vi "Calibration.vi"(0 "Mode":T3, 5 "Calib file":path, 9 "Simulate/Run":T2) -> (14 "Calib const":string[][](array[string]), 16 "Coefficients":dbl[][](array[numeric]) format="%.2f", 19 "Status Out":T1)   [LabVIEW 2021]
uses:
  Anemometry Sub Vis/Calibration/Calib_mode.ctl
  Anemometry Sub Vis/Controls/User_Specific_mode.ctl
  Anemometry Sub Vis/Gen Trav/Multi_Run_Status.ctl
  Anemometry Sub Vis/Controls/Post_Process.ctl
  Anemometry Sub Vis/Globals/Calib_global.vi
  Anemometry Sub Vis/Globals/Meas_global.vi
panel:
  in  "-ve Ref Values":bool
  out "String":string
  in  "poly fit order":i32=2 caption="Polynomial\nOrder" min=1 max=4 step=1
  out "Ref velocity":dbl[](array[numeric])=[2.4275346736, 2.4395664609, 2.453235235, 2.4247395837, 2.4277603784, 2.41169823, 2.4254144559, 2.424896502176921] format="%.3f"
  out "labels":string[](array[string])=["XW1 Volt", "XW2 Volt", "Entered Val", "Selector"]
  in  "Point selector 3":cluster{"Y":dbl, "X":dbl, "t/f":bool}[](array[cluster]) {"X" format="%#.2g"; "Y" format="%#.3f"}
  in  "n":dbl=0.45 format="%.4f"
  in  "Fixed n":bool=TRUE
  out "Sample of input signals":dbl[][](graph)
  in  "Sampling speeds":T4={"Samples/ch"=600, "Sample Rate/ch (Hz)"=100.0} {"Sample Rate/ch (Hz)" min=0; "Samples/ch" min=0 step=1}
  out "Calibration plot":cluster{cluster{dbl, dbl}[]}[](graph)
  in  "Point selector 4":T5(array[cluster]) {"Y2" format="%#.2f"; "X" format="%#.3f"; "Y" format="%#.2f"}
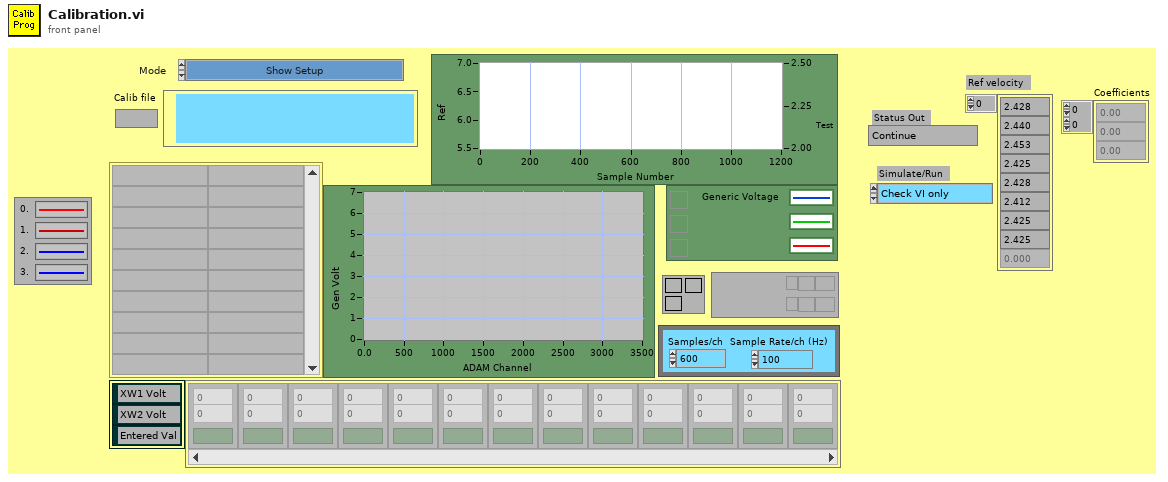
[diagram p1: front panel]
types:
  T1 = typedef "Multi_Run_Status.ctl" = enum16{"Continue", "Continue with Error", "Jump to Next Point", "Jump to Next Row", "Jump To Fall Back", "Terminate Run"}
  T2 = typedef "User_Specific_mode.ctl" = enum16{"Check VI only", "Run VI"}
  T3 = typedef "Calib_mode.ctl" = enum16{"Show Setup", "Take a New Calibration Point", "Refit Curve", "Setup Front Panel"}
  T4 = cluster{"Samples/ch":i32, "Sample Rate/ch (Hz)":sgl}
  T5 = cluster{"Y":dbl, "Y2":dbl, "X":dbl, "t/f":bool}[]
  T6 = typedef "Post_Process.ctl" = enum16{"Take New Data", "Post Process Raw Data File"}
  T7 = cluster{"Samples /ch":i32, "Sampling Rate /ch (Hz)":sgl}
  T8 = typedef "Ref_Inst_type.ctl" = enum16{"Propellor anemometer", "Pressure Transducer", "Raw voltage", "Pitot-static tube", "Generic Linear", "Generic Polynomial", "Thermocouple", "LDA", "Enter Value", "ADAM Channel"}
  T9 = typedef "Cal_Inst_type.ctl" = enum16{"Propeller anemometer", "Pressure Transducer", "Hot wire", "Cross wire velocity", "Cross wire angle", "Generic Linear", "Generic Polynomial", "Poly Fit Special", "Fast FID", "Thermocouple", "Cold wire", "Pulsed Wire"}
  T10 = cluster{"2nd Ref type":T8, "2nd inst present":bool}
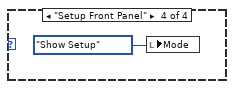
[diagram p4: hidden frame]
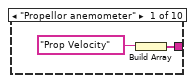
[diagram p8: hidden frame]
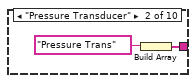
[diagram p9: hidden frame]
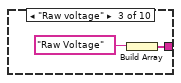
[diagram p10: hidden frame]
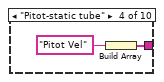
[diagram p11: hidden frame]
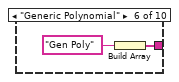
[diagram p12: hidden frame]
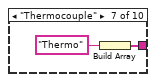
[diagram p13: hidden frame]
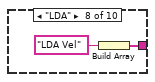
[diagram p14: hidden frame]
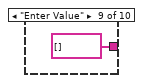
[diagram p15: hidden frame]
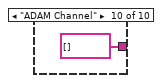
[diagram p16: hidden frame]
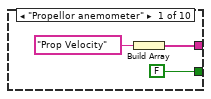
[diagram p17: hidden frame]
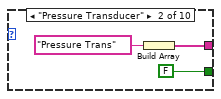
[diagram p18: hidden frame]
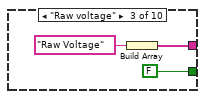
[diagram p19: hidden frame]
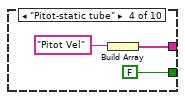
[diagram p20: hidden frame]
diagram:
  # "Temporary error bus for flow\ncontrol. No errors ever get\nwritten to it."
  n1 = flat-sequence {
    tunnel: "Simulate/Run" -> [w46]
    tunnel: errorcluster {"status"=FALSE, "code"=0, "source"=""} ("error constant") -> [w42]
    tunnel: [w42] -> w18
    frame #0 {
      w44 = FALSE  # Visible
      # "Calibration-Frame0"
      n2 = call "Run_EnFlo_Hub.vi"() -> ()  [unwired: 1 in, 7 out]
      n3 = case shown="\"Run VI\"" w46 {
        frame "Check VI only" {
        }
        frame "Run VI" {
          n4 = Current VI's Path() -> (path=w48:path)
          n5 = call "Open_Close_Front_Panel.ph.vi"("openWindow (T)"=TRUE ("Front Panel Window:Open"), "VI path"=w48) -> ()  [unwired: 1 in, 1 out]
        }
      }
      n6 = property on="String" class="Str"("Visible"=w44, "Blinking"=w44) -> ()  [unwired: 2 in, 2 out]
      n7 = global write "Calib_global.vi" "New Setup String"("") -> ()
      n8 = global write "Meas_global.vi" "Raw data option"(enum16{"Save raw data", "Raw data not saved"}."Save raw data" ("Raw data option")) -> ()
      n9 = global write "Meas_global.vi" "Post Process"(Post_Process."Take New Data" ("Post Process")) -> ()
    }
  }
  n10 = flat-sequence {
    tunnel: [w55] -> w2
    tunnel: [w54] -> w22
    tunnel: [w53] -> w38
    tunnel: w18 -> [w51]
    tunnel: [w51] -> w17
    tunnel: "Mode" -> [w50]
    frame #0 {
      # "Calibration-Frame1"
      n11 = call "Cal1-GetPath.vi"("Mode in"=w50, "Calib file"="Calib file") -> ("String output"=w53:string, "exists?"=w55:bool, "Path output"=w54:path)  [unwired: 7 in]
      n12 = local write "Calib file"(w54) -> ()
    }
  }
  n13 = flat-sequence {
    tunnel: [w63] -> w21
    tunnel: w22 -> [w62]
    tunnel: [w61] -> w36
    tunnel: [w60] -> w20
    tunnel: w17 -> [w59]
    tunnel: [w59] -> w16
    tunnel: "Mode" -> [w56]
    frame #0 {
      # "Calibration-Frame2"
      n14 = Current VI's Path() -> (path=w58:path)
      n15 = call "Running_as_top_level.vi"("Vi path name"=w58) -> ("Top Level"=w57:bool)  [unwired: 1 out]
      n16 = call "Cal2-GetMode.vi"("Calibration.vi running as top level VI?"=w57, "Mode in"=w56, "Path in"=w62) -> ("data mode"=w63:enum16{"Take new data point", "Refit Curve"}, "Mode out"=w60:T3, "Boolean"=w61:bool)  [unwired: 6 in]
    }
  }
  n17 = flat-sequence {
    tunnel: w21 -> [w68]
    tunnel: w20 -> [w67]
    tunnel: w36 -> [w65]
    tunnel: w16 -> [w64]
    tunnel: [w64] -> w15
    frame #0 {
      # "Calibration-Frame3"
      n18 = local read "Fixed n"() -> (w70:bool)
      n19 = call "Cal3-GetSetup.vi"("Sampling speeds"="Sampling speeds", "data mode"=w68, "Fixed n"=w70, "Mode in"=w67, "Boolean in"=w65) -> ("Sampling speeds Output"=w71:T7, "Fixed n out"=w69:bool, "Boolean out"=w66:bool)  [unwired: 4 in]
      n20 = case shown="True" w66 {
        tunnel: w71 -> [_ w74]
        tunnel: w69 -> [_ w73]
        frame False {
        }
        frame True {
          n21 = local write "Sampling speeds"(w74) -> ()
          n22 = local write "Fixed n"(w73) -> ()
        }
      }
    }
  }
  n23 = flat-sequence {
    tunnel: [w81] -> w39
    tunnel: [w80] -> w40
    tunnel: w22 -> [w79]
    tunnel: w2 -> [w78]
    tunnel: w38 -> [w77]
    tunnel: w15 -> [w76]
    tunnel: [w76] -> w14
    tunnel: "Mode" -> [w75]
    frame #0 {
      # "Calibration-Frame4"
      n24 = case shown="\"Setup Front Panel\"" w75 {
        frame Default {
        }
        frame "Setup Front Panel" {
          n25 = global read "Calib_global.vi" "Pre Setup String"() -> (w83:string)
          n26 = call "Get_value_from_string.vi"("Input string"=w83, "Variable name"="Polynomial Fit Order" ("Label for value")) -> ("Value"=w82:dbl)  [unwired: 1 in, 1 out]
          n27 = local write "poly fit order"(w82) -> ()
        }
      }
      n28 = call "Cal4-GetCalDataFrFile.vi"("StringName"=w77, "FileExists?"=w78, "CalibFilePath"=w79) -> ("CalibData"=w81:string, "HasData"=w80:bool)  [unwired: 7 in]
    }
  }
  n29 = flat-sequence {
    tunnel: w14 -> [w85]
    tunnel: [w85] -> w13
    frame #0 {
      w88 = ""
      # "Calibration-Frame5"
      n30 = global read "Calib_global.vi" "Ref Instrument type"() -> (w96:T8)
      n31 = global read "Calib_global.vi" "Instrument type"() -> (w99:T9)
      n32 = global read "Calib_global.vi" "2nd ref instrument"() -> (w95:T10)
      n33 = case shown="\"Generic Linear\"" w96 {
        tunnel: [w123 w126 w130 w132 w135 w138 w141 w144 string[] [] string[] []] -> w92
        tunnel: [FALSE FALSE FALSE FALSE FALSE FALSE FALSE FALSE FALSE FALSE] -> w87
        frame "Propellor anemometer" {
          n34 = Build Array("Prop Velocity") -> (w123:string[])
        }
        frame "Pressure Transducer" {
          n35 = Build Array("Pressure Trans") -> (w126:string[])
        }
        frame "Raw voltage" {
          n36 = Build Array("Raw Voltage") -> (w130:string[])
        }
        frame "Pitot-static tube" {
          n37 = Build Array("Pitot Vel") -> (w132:string[])
        }
        frame "Generic Linear" {
          n38 = Build Array("Gen Lin") -> (w135:string[])
        }
        frame "Generic Polynomial" {
          n39 = Build Array("Gen Poly") -> (w138:string[])
        }
        frame "Thermocouple" {
          n40 = Build Array("Thermo") -> (w141:string[])
        }
        frame "LDA" {
          n41 = Build Array("LDA Vel") -> (w144:string[])
        }
        frame "Enter Value" {
        }
        frame "ADAM Channel" {
        }
      }
      n42 = case shown="\"Thermocouple\"" w99 {
        tunnel: [w154 w158 w162 w166 w171 w176 w180 w184 w188 w192 w196 w201] -> w89
        tunnel: [FALSE FALSE FALSE FALSE FALSE FALSE TRUE TRUE FALSE FALSE TRUE TRUE] -> w91
        tunnel: [w152 w156 w160 w164 w169 w174 w178 w182 w186 w190 w194 FALSE] -> w86
        tunnel: w87 -> [w152 w156 w160 w164 w169 w174 w178 w182 w186 w190 w194 _]
        frame "Propeller anemometer" {
          n43 = Build Array("Prop Voltage") -> (w154:string[])
        }
        frame "Pressure Transducer" {
          n44 = Build Array("Pressure Trans") -> (w158:string[])
        }
        frame "Hot wire" {
          n45 = Build Array("HW Voltage") -> (w162:string[])
        }
        frame "Cross wire velocity" {
          n46 = Build Array("XW1 Voltage", "XW2 Voltage") -> (w166:string[])
        }
        frame "Cross wire angle" {
          n47 = Build Array("XW1 Voltage", "XW2 Voltage") -> (w171:string[])
        }
        frame "Generic Linear" {
          n48 = Build Array("Generic Voltage") -> (w176:string[])
        }
        frame "Generic Polynomial" {
          n49 = Build Array("Generic Voltage") -> (w180:string[])
        }
        frame "Poly Fit Special" {
          n50 = Build Array("Generic Voltage") -> (w184:string[])
        }
        frame "Fast FID" {
          n51 = Build Array("FF Voltage") -> (w188:string[])
        }
        frame "Thermocouple" {
          n52 = Build Array("Thermo Voltage") -> (w192:string[])
        }
        frame "Cold wire" {
          n53 = Build Array("CW Voltage") -> (w196:string[])
        }
        frame "Pulsed Wire" {
          n54 = local write "poly fit order"(3 ("polynomial order")) -> ()
          n55 = Build Array("PWA 1/TOF") -> (w201:string[])
        }
      }
      n56 = Unbundle By Name(w95) -> ("2nd Ref type"=w93:T8, "2nd inst present"=w94:bool)
      n57 = case shown="True" w94 {
        tunnel: w93 -> [_ w102]
        tunnel: [w101 w103] -> w90
        tunnel: w92 -> [w101 _]
        frame False {
        }
        frame True {
          n58 = case shown="\"Generic Linear\"" w102 {
            tunnel: [w104 w106 w109 w110 w112 w114 w116 w118 string[] [] string[] []] -> w103
            frame "Propellor anemometer" {
              n59 = Build Array("Prop Velocity") -> (w104:string[])
            }
            frame "Pressure Transducer" {
              n60 = Build Array("Pressure Trans") -> (w106:string[])
            }
            frame "Raw voltage" {
              n61 = Build Array("Raw Voltage") -> (w109:string[])
            }
            frame "Pitot-static tube" {
              n62 = Build Array("Pitot Vel") -> (w110:string[])
            }
            frame "Generic Linear" {
              n63 = Build Array("Gen Lin") -> (w112:string[])
            }
            frame "Generic Polynomial" {
              n64 = Build Array("Gen Poly") -> (w114:string[])
            }
            frame "Thermocouple" {
              n65 = Build Array("Thermo") -> (w116:string[])
            }
            frame "LDA" {
              n66 = Build Array("LDA Vel") -> (w118:string[])
            }
            frame "Enter Value" {
            }
            frame "ADAM Channel" {
            }
          }
        }
      }
      n67 = case shown="False" w86 {
        frame False {
          n68 = local write "-ve Ref Values"(FALSE ("-ve Ref Values")) -> ()
        }
        frame True {
        }
      }
      n69 = Build Array (concatenate)(w90, w89, w88, w88, w88) -> (w97:string[])
      n70 = property on="-ve Ref Values" class="Bool (strict)"("Visible"=w86) -> ()  [unwired: 2 in, 2 out]
      n71 = property on="poly fit order" class="DigNum (strict)"("Visible"=w91) -> ()  [unwired: 2 in, 2 out]
      n72 = for {
        N: 3 -> [_]
        tunnel: w97 -> [w150] mode=indexing
        i -> [w151]
        n73 = property on="Sample of input signals" class="WFGraph (strict)"("Active Plot"=w151, "Plot.Plot Name"=w150) -> ()  [unwired: 2 in, 2 out]
      }
    }
  }
  n74 = flat-sequence {
    tunnel: w13 -> [w203]
    tunnel: [w203] -> w12
    frame #0 {
      # "Calibration-Frame6"
      n75 = call "Cal6-MakeLabels.vi"() -> ("String"=w205:string, "String 2"=w206:string, "Boolean"=w204:bool, "Array"=→"labels":string[], "Boolean 2"=w208:bool, "Boolean 3"=w209:bool)  [unwired: 6 in]
      n76 = property on="Point selector 4" class="Arr (strict)"("Visible"=w208) -> ()  [unwired: 2 in, 2 out]
      n77 = property on="Calibration plot" class="XYGraph (strict)"("X Scale.Name Label.Text"=w206, "Y Scale.Name Label.Text"=w205) -> ()  [unwired: 2 in, 2 out]
      n78 = property on="n" class="DigNum (strict)"("Visible"=w204) -> ()  [unwired: 2 in, 2 out]
      n79 = property on="Fixed n" class="Bool (strict)"("Visible"=w204) -> ()  [unwired: 2 in, 2 out]
      n80 = property on="Point selector 3" class="Arr (strict)"("Visible"=w209) -> ()  [unwired: 2 in, 2 out]
    }
  }
  n81 = flat-sequence {
    tunnel: [w219] -> w35
    tunnel: [w218] -> w34
    tunnel: [w217] -> w33
    tunnel: [w216] -> w32
    tunnel: [w215] -> w31
    tunnel: [w214] -> w37
    tunnel: w39 -> [w213]
    tunnel: w40 -> [w212]
    tunnel: w38 -> [w211]
    tunnel: w12 -> [w210]
    tunnel: [w210] -> w11
    frame #0 {
      # "Calibration-Frame7"
      n82 = call "Cal7-GetCalNumbers.vi"("CalString"=w213, "StringName"=w211, "EarlierPoints"=w212) -> ("Array3"=w216:dbl[], "Array0"=w218:dbl[], "Array2"=w217:dbl[], "Array4"=w215:dbl[], "Array1"=w219:dbl[], "Array5"=w214:bool[])  [unwired: 3 in]
    }
  }
  n83 = flat-sequence {
    tunnel: w2 -> [w224]
    tunnel: w37 -> [w222]
    tunnel: w36 -> [w221]
    tunnel: w11 -> [w220]
    tunnel: [w220] -> w10
    frame #0 {
      # "Calibration-Frame8"
      n84 = And(x=w221, y=w224) -> (x .and. y?=w223:bool)
      n85 = case shown="True" w223 {
        tunnel: w222 -> [_ w225]
        frame False {
        }
        frame True {
          n86 = local read "Point selector 3"() -> (w229:cluster{"Y":dbl, "X":dbl, "t/f":bool}[])
          n87 = local read "Point selector 4"() -> (w226:T5)
          n88 = for {
            tunnel: w229 -> [w237]
            tunnel: [w239] -> w228 mode=indexing
            tunnel: w225 -> [w238] mode=indexing
            i -> [w236]
            n89 = Index Array(array=w237, index=w236) -> (element=w235:cluster{"Y":dbl, "X":dbl, "t/f":bool})
            n90 = Bundle By Name(cluster=w235, "t/f"=w238) -> (w239:cluster{"Y":dbl, "X":dbl, "t/f":bool})
          }
          n91 = for {
            tunnel: w226 -> [w232]
            tunnel: [w234] -> w227 mode=indexing
            tunnel: w225 -> [w233] mode=indexing
            i -> [w231]
            n92 = Index Array(array=w232, index=w231) -> (element=w230:cluster{"Y":dbl, "Y2":dbl, "X":dbl, "t/f":bool})
            n93 = Bundle By Name(cluster=w230, "t/f"=w233) -> (w234:cluster{"Y":dbl, "Y2":dbl, "X":dbl, "t/f":bool})
          }
          n94 = local write "Point selector 3"(w228) -> ()
          n95 = local write "Point selector 4"(w227) -> ()
        }
      }
    }
  }
  n96 = flat-sequence {
    tunnel: w20 -> [w241]
    tunnel: w10 -> [w240]
    tunnel: [w240] -> w9
    frame #0 {
      # "Calibration-Frame9"
      n97 = call "Cal9-GetInstSetup.vi"("Mode in"=w241) -> ()  [unwired: 11 in]
    }
  }
  n98 = flat-sequence {
    tunnel: w22 -> [w245]
    tunnel: [w244] -> w24
    tunnel: w9 -> [w243]
    tunnel: [w243] -> w8
    frame #0 {
      # "Calibration-Frame10"
      n99 = local read "poly fit order"() -> (w242:i32)
      n100 = call "Cal10-WriteOutCurrentSetup.vi"("poly fit order"=w242, "CalibrationPath"=w245) -> ("String"=w244:string)  [unwired: 9 in]
      n101 = call "Calib_read_files.vi"() -> ()  [unwired: 1 out]
    }
  }
  n102 = flat-sequence {
    tunnel: w35 -> [w264]
    tunnel: w34 -> [w263]
    tunnel: [w262] -> w30
    tunnel: [w261] -> w23
    tunnel: [w260] -> w29
    tunnel: w33 -> [w259]
    tunnel: w32 -> [w258]
    tunnel: [w257] -> w28
    tunnel: [w256] -> w27
    tunnel: w22 -> [w254]
    tunnel: w21 -> [w253]
    tunnel: w31 -> [w252]
    tunnel: w8 -> [w246]
    tunnel: [w246] -> w7
    frame #0 {
      # "These VI server references have been\nallowed temporarily to allow for further\nrefactoring of frame 11 to be \nrelatively straight forward."
      # "These VI server references have been\nallowed temporarily to allow for further\nrefactoring of frame 11 to be \nrelatively straight forward."
      # "Calibration-Frame11"
      n103 = control-ref of="String"() -> (w251:refnum<vi>)
      n104 = control-ref of="-ve Ref Values"() -> (w250:refnum<vi>)
      n105 = call "Cal11-RunMeasurement.vi"("String in"=w251, "reference in"=w250, "Results file output"=w254, "Din"=w258, "CIn"=w263, "EIn"=w252, "BIn"=w259, "data mode"=w253, "Ain"=w264, "-ve Ref Values"="-ve Ref Values") -> ("Aout"=w261:dbl[], "BOut"=w260:dbl[], "Status Out"=→"Status Out":T1, "COut"=w262:dbl[], "Dout"=w257:dbl[], "EOut"=w256:dbl[], "String"=→"String":string, "Sample of input signals"=→"Sample of input signals":dbl[][])  [unwired: 2 in]
    }
  }
  n106 = flat-sequence {
    tunnel: w23 -> [w272]
    tunnel: w29 -> [w271]
    tunnel: w27 -> [w270]
    tunnel: w30 -> [w269]
    tunnel: [w268] -> w26
    tunnel: w28 -> [w267]
    tunnel: [w266] -> w25
    tunnel: [w265] -> w6
    tunnel: w7 -> [w265]
    frame #0 {
      # "Calibration-Frame12"
      n107 = call "Calibration-Frame12.vi"("Din"=w267, "Ein"=w270, "CsortBy"=w269, "Bin"=w271, "Ain"=w272) -> ("ArrayCABDE"=w268:dbl[][], "Sort Index"=w266:i32[])  [unwired: 5 in]
      "Ref velocity" <- w267
    }
  }
  n108 = flat-sequence {
    tunnel: w22 -> [w291]
    tunnel: w25 -> [w290]
    tunnel: w26 -> [w275]
    tunnel: w6 -> [w273]
    tunnel: [w273] -> w5
    frame #0 {
      w282 = FALSE  # t/f
      w283 = FALSE  # t/f
      # "Calibration-Frame13"
      n109 = Index Array(array="Point selector 3", index=0) -> (element=w288:cluster{"Y":dbl, "X":dbl, "t/f":bool})
      n110 = Index Array(array="Point selector 4", index=0) -> (element=w280:cluster{"Y":dbl, "Y2":dbl, "X":dbl, "t/f":bool})
      n111 = Bundle By Name(cluster=w288, "t/f"=w283) -> (w284:cluster{"Y":dbl, "X":dbl, "t/f":bool})
      n112 = Bundle By Name(cluster=w280, "t/f"=w282) -> (w281:cluster{"Y":dbl, "Y2":dbl, "X":dbl, "t/f":bool})
      n113 = Build Array (concatenate)("Point selector 3", w284) -> (w286:cluster{"Y":dbl, "X":dbl, "t/f":bool}[])
      n114 = Build Array (concatenate)("Point selector 4", w281) -> (w277:T5)
      n115 = for {
        tunnel: w286 -> [w303]
        tunnel: w290 -> [w300] mode=indexing
        tunnel: [w302] -> w287 mode=indexing
        tunnel: w277 -> [w301]
        tunnel: [w299] -> w276 mode=indexing
        n116 = Index Array(array=w303, index=w300) -> (element=w302:cluster{"Y":dbl, "X":dbl, "t/f":bool})
        n117 = Index Array(array=w301, index=w300) -> (element=w299:cluster{"Y":dbl, "Y2":dbl, "X":dbl, "t/f":bool})
      }
      n118 = call "Calib_Analyse_fit.vi"("Calib file"=w291, "Input points"=w275, "polynomial order"="poly fit order", "Fixed n"="Fixed n", "n"="n", "Point selector 3"=w287, "Point selector 4"=w276) -> ("Calib const"=→"Calib const":string[][], "Calibration plot"=→"Calibration plot":cluster{cluster{dbl, dbl}[]}[], "Point selector 3 out"=w296:cluster{"Y":dbl, "X":dbl, "t/f":bool}[], "Coefficients"=→"Coefficients":dbl[][], "Point selector 4 out"=w295:T5)  [unwired: 4 out]
      n119 = local write "Point selector 3"(w296) -> ()
      n120 = local write "Point selector 4"(w295) -> ()
    }
  }
  n121 = flat-sequence {
    tunnel: w24 -> [w306]
    tunnel: w22 -> [w305]
    tunnel: w5 -> [w304]
    tunnel: [w304] -> w4
    frame #0 {
      # "Calibration-Frame14"
      n122 = call "Calibration-Frame14.vi"("Results file output"=w305, "String"=w306) -> ()  [unwired: 10 in]
    }
  }
  n123 = flat-sequence {
    tunnel: w21 -> [w312]
    tunnel: w22 -> [w311]
    tunnel: w23 -> [w310]
    tunnel: w4 -> [w309]
    tunnel: [w309] -> w3
    frame #0 {
      # "Calibration-Frame15"
      n124 = Current VI's Path() -> (path=w308:path)
      n125 = call "Running_as_top_level.vi"("Vi path name"=w308) -> ("Top Level"=w307:bool)  [unwired: 1 out]
      n126 = call "Calibration-Frame15.vi"("Reset Measurement Prog"=w307, "Array 8"=w310, "data mode"=w312, "Results file output"=w311) -> ()  [unwired: 8 in]
    }
  }
  n127 = flat-sequence {
    tunnel: w20 -> [w313]
    tunnel: w3 -> [_]
    frame #0 {
      # "Calibration-Frame16"
      n128 = case shown="\"Show Setup\"" w313 {
        frame "Show Setup" {
          n129 = local write "Mode"(Calib_mode."Take a New Calibration Point" ("Mode")) -> ()
        }
        frame "Take a New Calibration Point" {
        }
        frame "Refit Curve" {
        }
        frame "Setup Front Panel" {
          n130 = local write "Mode"(Calib_mode."Show Setup" ("Mode")) -> ()
        }
      }
      n131 = global write "Calib_global.vi" "Calibration Points"(dbl[] [] ("Calibration Points")) -> ()
    }
  }
